vi "ActionVIOnCompile.vi"(8 "error in (no error)":errorcluster, 11 "Device Item Ref in":T1 format="%.0x") -> (0 "error out":errorcluster)   [LabVIEW 2020, in "gRPC Data Server System Explorer.lvlib"]
uses:
  gRPC Data Server System Explorer.lvlib
  <vilib>/NI VeriStand/Custom Device API/Custom Device Item Ref.ctl
  Shared/Compiled.Settings.ctl
  <vilib>/NI VeriStand/Custom Device API/Set Item Property (Variant).vi
  <vilib>/NI VeriStand/Custom Device Tools/Custom Device Utility Library/Custom Device Utility Library.lvlib
  <vilib>/NI VeriStand/Custom Device Tools/Custom Device Utility Library/NI VeriStand - Search for Item by Name.vi
  <vilib>/NI VeriStand/Custom Device API/Custom Device API.lvlib
  <vilib>/NI/NIVS Inline Async API/_Data Access System Explorer/Data Access System Explorer.lvlib
  Shared/gRPC Data Server Shared.lvlib
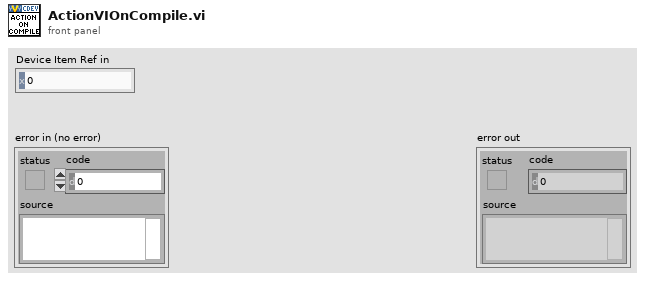
[diagram p1: front panel]
types:
  T1 = typedef "Custom Device API.lvlib/Custom Device Item Ref.ctl" = u64
  T2 = cluster{"Name":string, "Type":enum16{"Output/Write", "Input/Read", "Input/ReadWrite"}, "VS Refs":T1[]}
  T3 = enum16{"Output/Write", "Input/Read", "Input/ReadWrite"}
  T4 = typedef "gRPC Data Server Shared.lvlib/Compiled.Settings.ctl" = cluster{"Name":string, "Server Address":string, "Async?":bool, "Key File":path, "Cert File":path, "Channel Name":string[], "Initial Value":string[]}
  T5 = typedef "Custom Device API.lvlib/Custom Device Item Info.ctl" = cluster{"Name":string, "Is Channel":bool, "GUID":string, "Is Waveform":bool}
  T6 = cluster{"Name":string, "Type":enum16{"Output/Write", "Input/Read", "Input/ReadWrite"}, "VS Refs":T1[]}[]
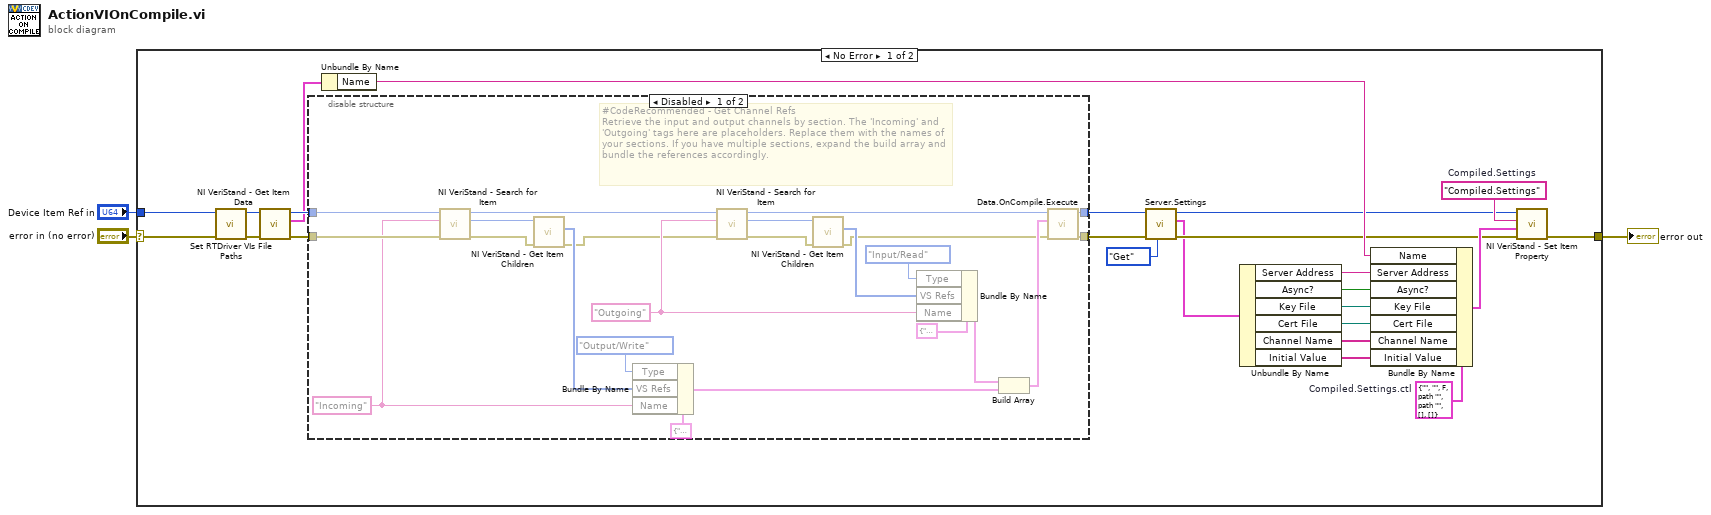
[diagram p0: block diagram]
diagram:
  n1 = case shown="No Error" "error in (no error)" {
    selector: "error in (no error)" -> [w6 w53]
    tunnel: [w25 w53] -> w2
    tunnel: "Device Item Ref in" -> [w7 _]
    frame No Error {
      w20 = T4 {"Name"="", "Server Address"="", "Async?"=FALSE, "Key File"=path "", "Cert File"=path "", "Channel Name"=[], "Initial Value"=[]}  # Compiled.Settings.ctl
      w27 = "Compiled.Settings"  # Compiled.Settings
      n2 = call "Set RTDriver VIs File Paths.vi"("error in (no error)"=w6, "Item Ref in"=w7) -> ("error out"=w4:errorcluster, "Item Ref out"=w5:T1)  [unwired: 8 in]
      n3 = call <vilib>:"NI VeriStand - Get Item Data.vi"("error in (no error)"=w4, "Item Ref in"=w5) -> ("error out"=w23:errorcluster, "Item Info"=w22:T5, "Item Ref out"=w24:T1)  [unwired: 6 in, 1 out]
      n4 = disable-structure shown="Disabled" {
        disable-tunnel: w24 -> [w46 w52]
        disable-tunnel: w23 -> [w45 w51]
        disable-tunnel: [w29 w51] -> w18
        disable-tunnel: [w28 w52] -> w19
        frame Disabled {
          w42 = "Outgoing" ("Item Name")
          w44 = "Incoming" ("Item Name")
          # "#CodeRecommended - Get Channel Refs\nRetrieve the input and output channels by section. The 'Incoming' and 'Outgoing' tags here are placeholders. Replace them with the names of your sections. If you have multiple sections, expand the build array and bundle the references accordingly."
          n5 = call-poly <vilib>:"NI VeriStand - Search for Item.vi"("error in"=w45, "Item Name"=w44, "Section Ref in"=w46) -> ("error out"=w50:errorcluster, "Item Ref"=w49:T1, "Section Ref out"=w31:T1)  [unwired: 5 in, 1 out]
          n6 = call <vilib>:"NI VeriStand - Get Item Children.vi"("error in (no error)"=w50, "Item Ref in"=w49) -> ("error out"=w30:errorcluster, "Child Refs"=w43:T1[])  [unwired: 6 in, 2 out]
          n7 = Bundle By Name(cluster=T2 {"Name"="", "Type"=enum."Output/Write", "VS Refs"=[]} ("Group"), "Type"=T3."Output/Write", "VS Refs"=w43, "Name"=w44) -> (w34:T2)
          n8 = call-poly <vilib>:"NI VeriStand - Search for Item.vi"("error in"=w30, "Item Name"=w42, "Section Ref in"=w31) -> ("error out"=w47:errorcluster, "Item Ref"=w48:T1, "Section Ref out"=w32:T1)  [unwired: 5 in, 1 out]
          n9 = call <vilib>:"NI VeriStand - Get Item Children.vi"("error in (no error)"=w47, "Item Ref in"=w48) -> ("error out"=w33:errorcluster, "Child Refs"=w38:T1[])  [unwired: 6 in, 2 out]
          n10 = Bundle By Name(cluster=T2 {"Name"="", "Type"=enum."Output/Write", "VS Refs"=[]} ("Group"), "Type"=T3."Input/Read", "VS Refs"=w38, "Name"=w42) -> (w40:T2)
          n11 = Build Array(w40, w34) -> (w37:T6)
          n12 = call <vilib>:"Data.OnCompile.Execute.vi"("error in"=w33, "VS Ref Groups"=w37, "Custom Device Ref"=w32) -> ("error out"=w29:errorcluster, "Custom Device Ref"=w28:T1)  [unwired: 7 in]
        }
        frame Enabled {
        }
      }
      n13 = Unbundle By Name(w22) -> ("Name"=w21:string)
      n14 = call "Server.Settings.vi"("Action"=enum8{"Get", "Set"}."Get", "error in (no error)"=w18, "Parent Ref in"=w19) -> ("error out"=w16:errorcluster, "Client Settings Out"=w14:T4, "Item Ref out"=w17:T1)  [unwired: 6 in]
      n15 = Unbundle By Name(w14) -> ("Server Address"=w13:string, "Async?"=w12:bool, "Key File"=w11:path, "Cert File"=w10:path, "Channel Name"=w9:string[], "Initial Value"=w8:string[])
      n16 = Bundle By Name(cluster=w20, "Name"=w21, "Server Address"=w13, "Async?"=w12, "Key File"=w11, "Cert File"=w10, "Channel Name"=w9, "Initial Value"=w8) -> (w26:T4)
      n17 = call-poly <vilib>:"NI VeriStand - Set Item Property.vi"("error in (no error)"=w16, "Value"=w26, "Property Name"=w27, "Item Ref in"=w17) -> ("error out"=w25:errorcluster)  [unwired: 5 in, 2 out]
    }
    frame Error {
    }
  }
  "error out" <- w2
